vi "Close.vi"(8 "error in":errorcluster, 11 "Series Base in":refnum<class "Series Base.lvclass">) -> (0 "error out":errorcluster, 3 "Series Base out":refnum<class "Series Base.lvclass">)   [LabVIEW 2023, in "HAL GOOP4.lvlib" / "Series Base.lvclass"]
uses:
  Series Base.lvclass
  Series Base.lvclass/Series Base.ctl
  Measure and Stimulus Subsystems/Measure and Stimulus Subsystems.lvclass
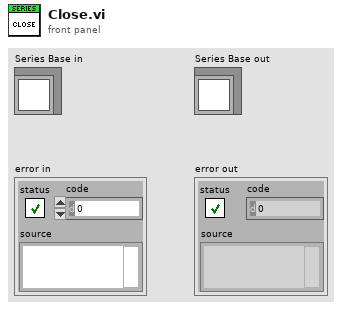
[diagram p1: front panel]
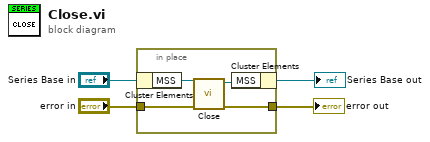
[diagram p0: block diagram]
diagram:
  n1 = in-place "In Place Element Structure" {
    in-place-border: "error in" -> [w6]
    in-place-border: [w5] -> w2
    n2 = in-place-cluster #1("Series Base in") -> ("MSS"=w8:refnum<class "Measure and Stimulus Subsystems.lvclass">)
    n3 = call "Close.vi"("error in"=w6, "MSS in"=w8) -> ("error out"=w5:errorcluster, "MSS out"=w7:refnum<class "Measure and Stimulus Subsystems.lvclass">)  [unwired: 8 in]
    n4 = in-place-cluster #1("MSS"=w7) -> (→"Series Base out":refnum<class "Series Base.lvclass">)
  }
  "error out" <- w2
